vi "子界面-生成检测结果和报告-9.23测试版.vi"(0 "Particle Measurements (Pixels)":dbl[][](array[numeric]) format="%.2f", 1 "面积 (pixels)":i32, 2 "框号":i64, 3 "产品序号":string, 4 "测试人":string) -> (5 "?":bool=TRUE)   [LabVIEW 2018]
uses:
  <vilib>/Utility/NIReport.llb/Report Type.ctl
  <vilib>/Utility/NIReport.llb/Append Report Text (str wrap).vi
  <vilib>/addons/_office/word.llb/Word Edit Cell ([dbl]).vi
  <vilib>/Utility/NIReport.llb/NI_report.lvclass
  <vilib>/addons/_office/NI_ReportGenerationToolkit.lvlib
  <vilib>/Utility/NIReport.llb/NI_ReportGenerationCore.lvlib
  <vilib>/Utility/NIReport.llb/Word/NI_Word.lvclass
panel:
  in  "格式字符串":string="%f"
  in  "分隔符（'\\'代码显示）":string="\t"
  out "所选区域检测结果":string[][](table)
  out "报告生成路径":path
  out "所选区域信息":string
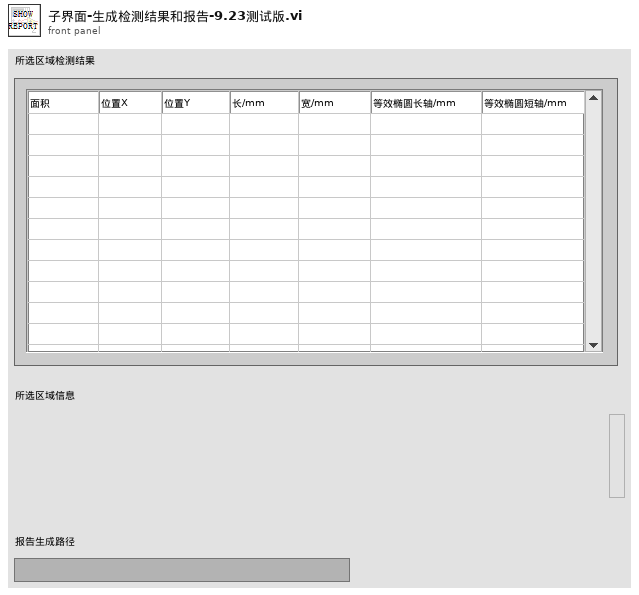
[diagram p1: front panel]
types:
  T1 = cluster{"position (Excel)":cluster{"row":i32, "column":i32}, "name (Excel)":string, "bookmark (Word)":string}
  T2 = typedef "NI_ReportGenerationCore.lvlib/Report Type.ctl" = enum16{"HTML", "Word", "Excel"}
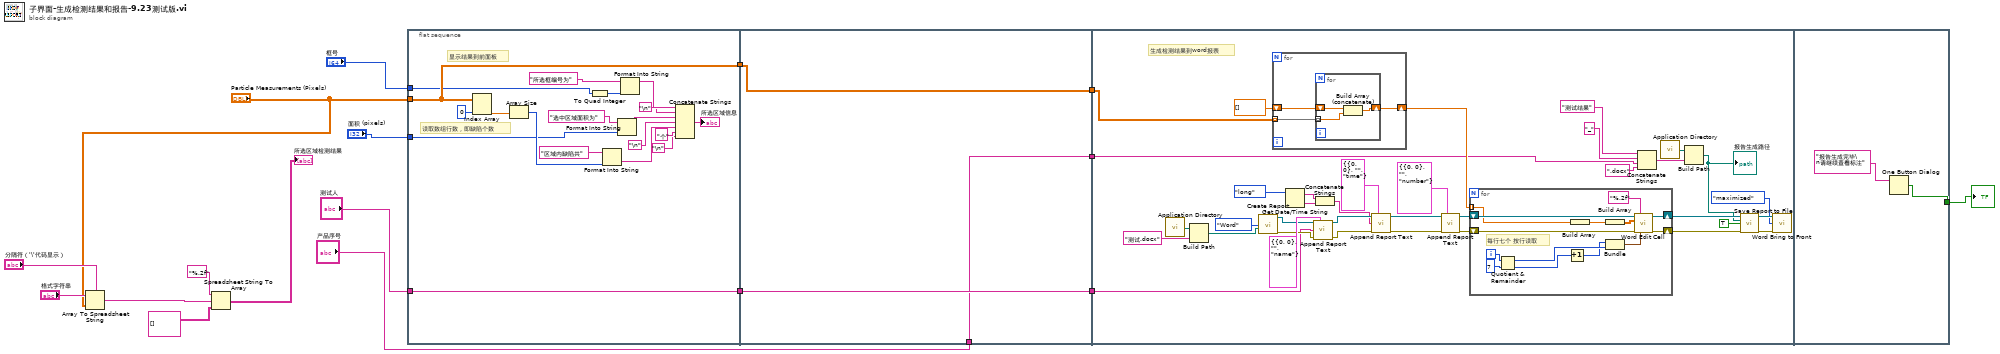
[diagram p0: block diagram]
diagram:
  n1 = Array To Spreadsheet String(delimiter (Tab)="分隔符（'\\'代码显示）", array="Particle Measurements (Pixels)", 3:"格式字符串") -> (spreadsheet string=w5:string)
  n2 = Spreadsheet String To Array(format string="%.2f", spreadsheet string=w5, array type (2D Dbl)=string[][] [] ("Array")) -> (array=→"所选区域检测结果":string[][])  [unwired: 1 in]
  n3 = flat-sequence {
    tunnel: "Particle Measurements (Pixels)" -> [w21]
    tunnel: [w21] -> w17
    tunnel: "面积 (pixels)" -> [w20]
    tunnel: "框号" -> [w19]
    tunnel: [w18] -> w11
    tunnel: "测试人" -> [w18]
    tunnel: w17 -> [w37]
    tunnel: [w37] -> w16
    tunnel: [w39] -> w12
    tunnel: w11 -> [w39]
    tunnel: [w38] -> w9
    tunnel: "产品序号" -> [w38]
    tunnel: w16 -> [w42]
    tunnel: w12 -> [w41]
    tunnel: w9 -> [w40]
    tunnel: [w96] -> w14
    frame #0 {
      # "显示结果到前面板"
      # "读取数组行数，即缺陷个数"
      n4 = Index Array(array=w21, index (col)=0 ("禁用的索引 (列)")) -> (element=w30:dbl[])  [unwired: 1 in]
      n5 = Array Size(array=w30) -> (size(s)=w32:i32)
      n6 = To Quad Integer(1:w19) -> (0:w33:i64)
      n7 = Format Into String(initial string="区域内缺陷共" ("初始字符串"), w32) -> (resulting string=w35:string)  [unwired: 2 in, 1 out]
      n8 = Format Into String(initial string="选中区域面积为" ("字符串"), w20) -> (resulting string=w36:string)  [unwired: 2 in, 1 out]
      n9 = Format Into String(initial string="所选框编号为" ("初始字符串"), w33) -> (resulting string=w34:string)  [unwired: 2 in, 1 out]
      n10 = Concatenate Strings(w34, "\n", w36, "\n", w35, "个" ("字符串"), "\n") -> (→"所选区域信息":string)
    }
    frame #1 {
    }
    frame #2 {
      # "生成检测结果到word报表"
      n11 = call <vilib>:"Application Directory.vi"() -> ("Application Directory"=w43:path)
      n12 = Build Path(base path=w43, name or relative path="测试.docx") -> (appended path=w46:path)
      n13 = call <vilib>:"Create Report.vi"("report type"=Report_Type."Word" ("Report Type"), "template (empty)"=w46) -> ("report out"=w71:refnum<class "NI_report.lvclass">, "error out"=w74:errorcluster)  [unwired: 12 in]
      n14 = for {
        tunnel: w42 -> [w78] mode=indexing
        shift-right: [w76] -> w70
        shift-left: dbl[] [] ("元素") -> [w77]
        n15 = for {
          tunnel: w78 -> [w81] mode=indexing
          shift-right: [w79] -> w76
          shift-left: w77 -> [w80]
          n16 = Build Array (concatenate)(w80, w81) -> (w79:dbl[])
        }
      }
      n17 = Get Date/Time String(date format (0)=enum16{"short", "long", "abbreviated"}."long" ("日期格式(0)")) -> (date string=w47:string, time string=w49:string)  [unwired: 2 in]
      n18 = call-poly <vilib>:"Append Report Text.vi"("report in"=w71, "MS Office parameters"=T1 {"position (Excel)"={"row"=0, "column"=0}, "name (Excel)"="", "bookmark (Word)"="name"}, "text"=w41, "error in (no error)"=w74) -> ("report out"=w72:refnum<class "NI_report.lvclass">, "error out"=w73:errorcluster)  [unwired: 8 in, 2 out]
      n19 = Concatenate Strings(w47, w49) -> (w48:string)
      n20 = call-poly <vilib>:"Append Report Text.vi"("report in"=w72, "MS Office parameters"=T1 {"position (Excel)"={"row"=0, "column"=0}, "name (Excel)"="", "bookmark (Word)"="time"}, "text"=w48, "error in (no error)"=w73) -> ("report out"=w63:refnum<class "NI_report.lvclass">, "error out"=w64:errorcluster)  [unwired: 8 in, 2 out]
      n21 = call-poly <vilib>:"Append Report Text.vi"("report in"=w63, "MS Office parameters"=T1 {"position (Excel)"={"row"=0, "column"=0}, "name (Excel)"="", "bookmark (Word)"="number"}, "error in (no error)"=w64) -> ("report out"=w65:refnum<class "NI_report.lvclass">, "error out"=w66:errorcluster)  [unwired: 9 in, 2 out]
      n22 = for {
        shift-right: [w95] -> w67
        shift-left: w65 -> [w90]
        shift-right: [w94] -> w68
        shift-left: w66 -> [w89]
        tunnel: w70 -> [w83] mode=indexing
        i -> [w91]
        # "每行七个 按行读取"
        n23 = Quotient & Remainder(x=w91, y=7) -> (x-y*floor(x/y)=w88:i32, floor(x/y)=w87:i32)
        n24 = Increment(x=w87) -> (x+1=w86:i32)
        n25 = Build Array(w83) -> (w85:dbl[])
        n26 = Build Array(w85) -> (w84:dbl[][])
        n27 = Bundle(w86, w88) -> (w93:cluster{i32, i32})  [unwired: 1 in]
        n28 = call-poly <vilib>:"Word Edit Cell.vi"("report in"=w90, "format string (%.3f)"="%.2f", "value"=w84, "error in (no error)"=w89, "start (0, 0)"=w93) -> ("report out"=w95:refnum<class "NI_report.lvclass">, "error out"=w94:errorcluster)  [unwired: 9 in]
      }
      n29 = Concatenate Strings("测试结果" ("字符串"), "_" ("名称或相对路径"), w40, ".docx" ("名称或相对路径")) -> (w55:string)
      n30 = call <vilib>:"Application Directory.vi"() -> ("Application Directory"=w54:path)
      n31 = Build Path(base path=w54, name or relative path=w55) -> (appended path=w53:path)
      "报告生成路径" <- w53
      n32 = call-dynamic "Save Report to File.vi"("report in"=w67, "report file path"=w53, "prompt to replace? (F)"=TRUE, "error in (no error)"=w68) -> ("report out"=w60:refnum<class "NI_report.lvclass">, "error out"=w61:errorcluster)  [unwired: 10 in]
      n33 = call <vilib>:"Word Bring to Front.vi"("report in"=w60, "window state (maximized)"=enum16{"maximized", "minimized", "normal"}."maximized", "error in (no error)"=w61) -> ()  [unwired: 11 in, 2 out]
    }
    frame #3 {
      n34 = One Button Dialog(message="报告生成完毕\n请继续查看标注" ("消息")) -> (true=w96:bool)  [unwired: 1 in]
    }
  }
  "?" <- w14
